vi "Get all divisors-exhaustive enumeration.vi"(8 "error in (no error)":errorcluster, 11 "x":i32) -> (0 "error out":errorcluster, 1 "Execution time (ms)-Total":u32, 2 "no. of divisors":i32, 3 "Divisors":i32[](array[numeric]))   [LabVIEW 2021, in "Numeric Utilities.lvlib"]
uses:
  Numeric Utilities.lvlib
  Named Timers/Named Timers.lvlib
panel:
  out "Loop iteration":i32
  # "Development\ncontrols/indicators useful for development and testing, but which are not outputs of the VI"
  # "Input\nInputs to the VI"
  # "Output\nOutputs of the VI"
  # "Description\n\nBlank VI with error handling case. \n\nSummarize the use of this VI in this space."
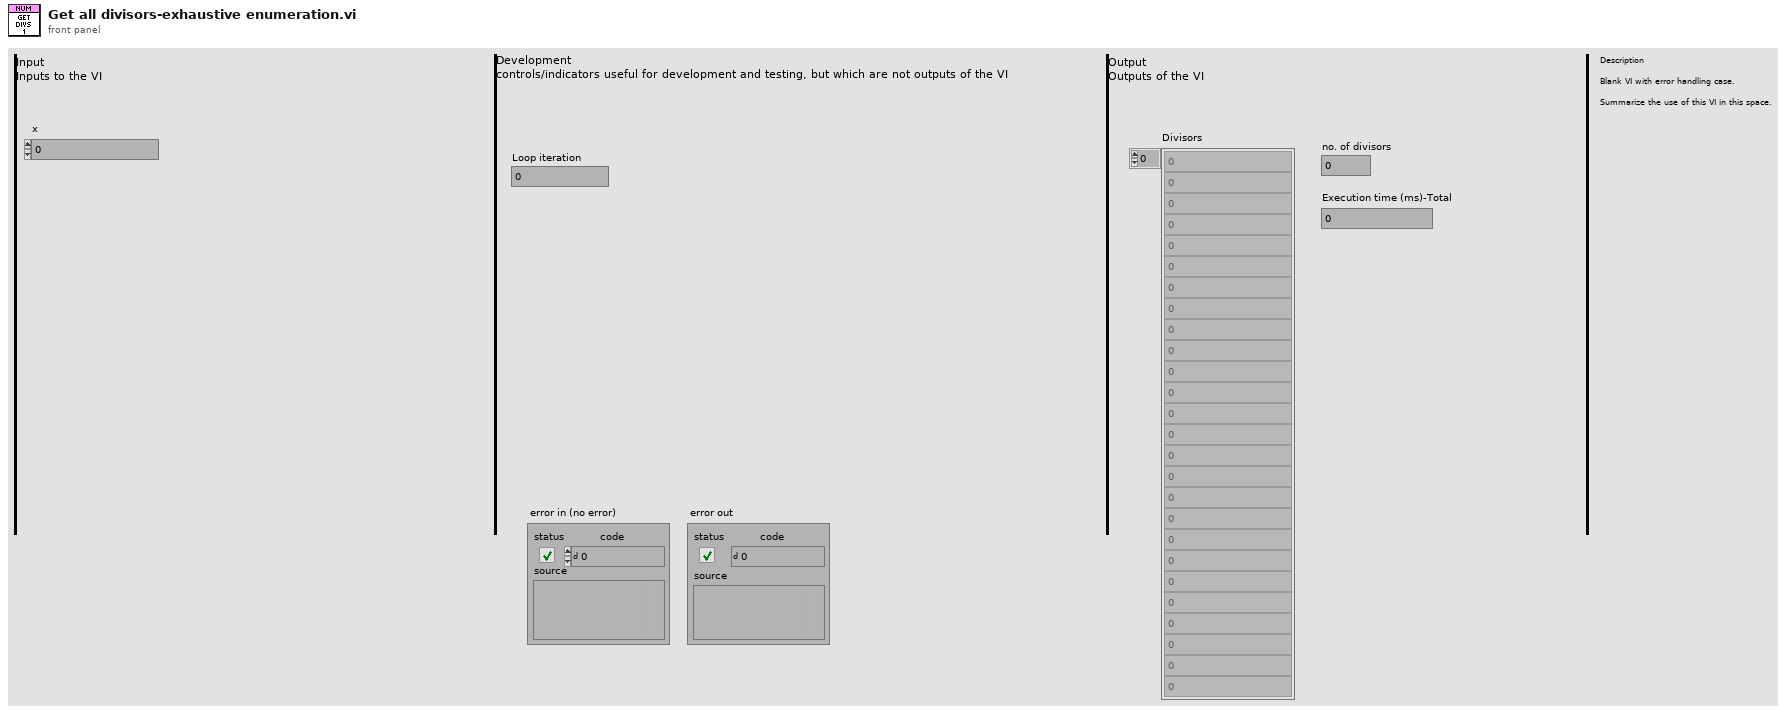
[diagram p1: front panel]
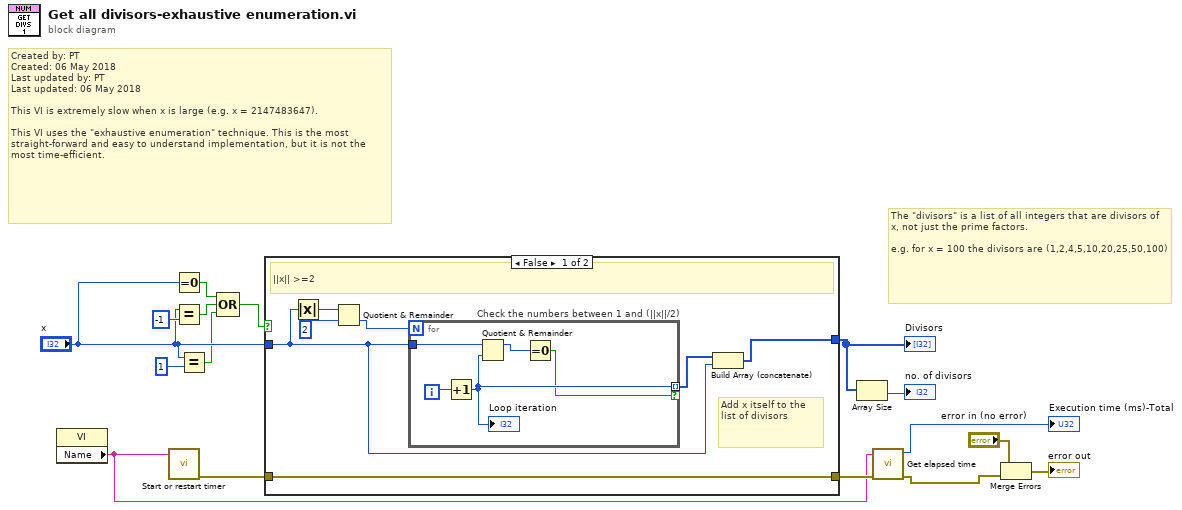
[diagram p0: block diagram]
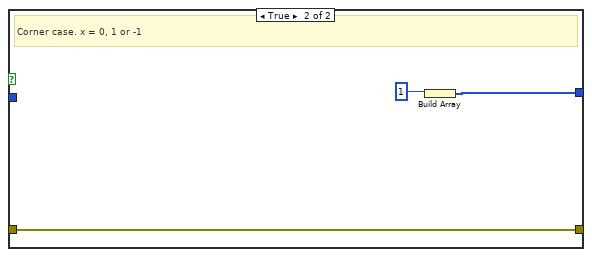
[diagram p2: hidden frame]
diagram:
  # "The \"divisors\" is a list of all integers that are divisors of x, not just the prime factors.\n\ne.g. for x = 100 the divisors are (1,2,4,5,10,20,25,50,100)"
  # "Created by: PT\nCreated: 06 May 2018\nLast updated by: PT\nLast updated: 06 May 2018\n\nThis VI is extremely slow when x is large (e.g. x = 2147483647).\n\nThis VI uses the \"exhaustive enumeration\" technique. This is the most straight-forward and easy to understand implementation, but it is not the most time-efficient."
  n1 = property class="VI"() -> ("Name"=w4:string)  [unwired: 2 in, 2 out]
  n2 = call "Start or restart timer.vi"("Timer name"=w4) -> ("error out"=w6:errorcluster)  [unwired: 10 in]
  n3 = Equal To 0?(x="x") -> (x = 0?=w15:bool)
  n4 = Equal?(x="x", y=-1) -> (x = y?=w10:bool)
  n5 = Equal?(x="x", y=1) -> (x = y?=w11:bool)
  n6 = Compound Arithmetic op=OR(w15, w10, w11) -> (w16:bool)
  n7 = case shown="False" w16 {
    tunnel: "x" -> [w19 _]
    tunnel: [w20 w29] -> w9
    tunnel: w6 -> [w17 w31]
    tunnel: [w17 w31] -> w5
    frame False {
      # "Add x itself to the list of divisors"
      # "||x|| >=2"
      n8 = Absolute Value(x=w19) -> (abs(x)=w18:i32)
      n9 = Quotient & Remainder(x=w18, y=2) -> (floor(x/y)=w22:i32)  [unwired: 1 out]
      n10 = for "Check the numbers between 1 and (||x||/2)" {
        N: w22 -> [_]
        tunnel: w19 -> [w28]
        tunnel: [w25] -> w21 mode=indexing if=w24
        i -> [w26]
        n11 = Increment(x=w26) -> (x+1=w25:i32)
        "Loop iteration" <- w25
        n12 = Quotient & Remainder(x=w28, y=w25) -> (x-y*floor(x/y)=w27:i32)  [unwired: 1 out]
        n13 = Equal To 0?(x=w27) -> (x = 0?=w24:bool)
      }
      n14 = Build Array (concatenate)(w21, w19) -> (w20:i32[])
    }
    frame True {
      # "Corner case. x = 0, 1 or -1"
      n15 = Build Array(1) -> (w29:i32[])
    }
  }
  "Divisors" <- w9
  n16 = Array Size(array=w9) -> (size(s)=→"no. of divisors":i32)
  n17 = call "Get elapsed time.vi"("error in (no error)"=w5, "Timer name"=w4) -> ("error out"=w2:errorcluster, "Elapsed time (ms)"=→"Execution time (ms)-Total":u32)  [unwired: 6 in, 2 out]
  n18 = Merge Errors("error in (no error)", w2) -> (→"error out":errorcluster)
